vi "Read Attributes.vi"(8 "error in (no error)":errorcluster, 11 "Element-XML in":refnum<class "Element-XML.lvclass">) -> (0 "error out":errorcluster, 2 "Attributes":refnum<class "Attribute-XML.lvclass">[](array[class]), 3 "Element-XML out":refnum<class "Element-XML.lvclass">)   [LabVIEW 2013, in "MaterialCharacterization.lvlib" / "Element-XML.lvclass"]
uses:
  Element-XML.lvclass
  Attribute-XML/Attribute-XML.lvclass
  Element-XML.lvclass/Element-XML.ctl
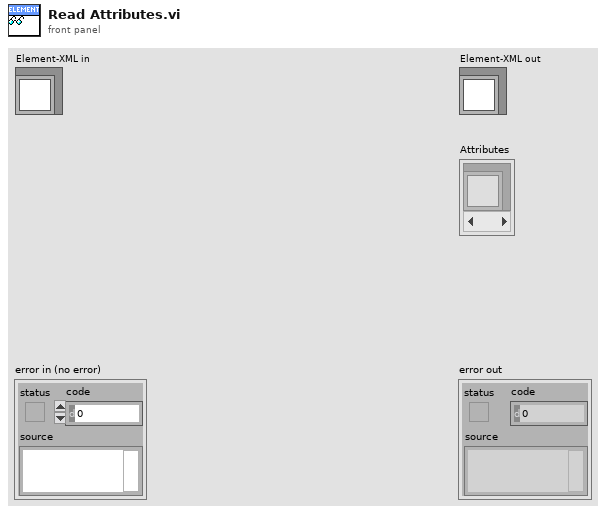
[diagram p1: front panel]
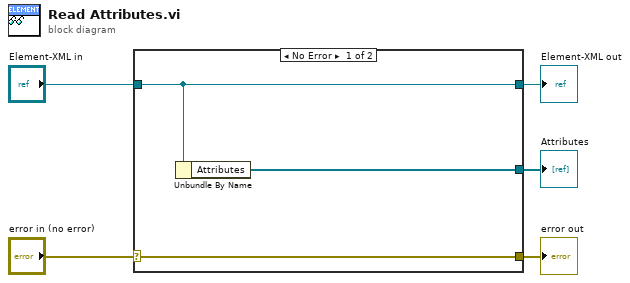
[diagram p0: block diagram]
diagram:
  n1 = case shown="No Error" "error in (no error)" {
    selector: "error in (no error)" -> [w8 w9]
    tunnel: [w8 w9] -> w4
    tunnel: [w7 w10] -> w2
    tunnel: "Element-XML in" -> [w7 w10]
    tunnel: [w6 _] -> w1
    frame No Error {
      n2 = Unbundle By Name(w7) -> ("Attributes"=w6:refnum<class "Attribute-XML.lvclass">[])
    }
    frame Error {
    }
  }
  "error out" <- w4
  "Element-XML out" <- w2
  "Attributes" <- w1
